vi "Door Poka Yoke_UI.vi"(8 "error in (no error)":errorcluster, 10 "Door Poka Yoke":bool, 11 "JSON FilePath":path) -> (0 "error out":errorcluster)   [LabVIEW 2019, in "ZenGage v3.0 UI.lvclass"]
uses:
  ZenGage v3.0 UI.lvclass
panel:
  out "Time taken":u32
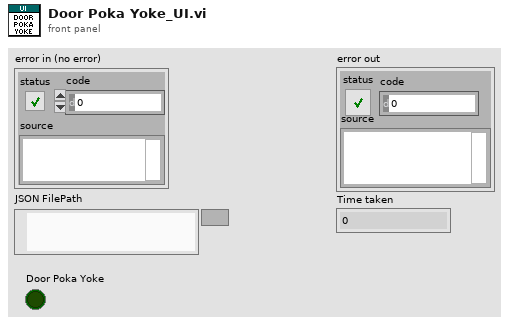
[diagram p1: front panel]
types:
  T1 = enum16{"Action Failed", "Append", "Insert", "Replace"}
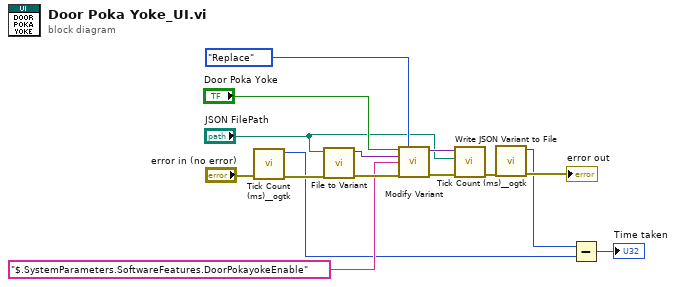
[diagram p0: block diagram]
diagram:
  n1 = call <userlib>:"Tick Count (ms)__ogtk.vi"("error in (no error)"="error in (no error)") -> ("error out"=w6:errorcluster, "millisecond timer value"=w2:u32)  [unwired: 9 in]
  n2 = call <vilib>:"File to Variant.vi"("JSON FilePath"="JSON FilePath", "error in (no error)"=w6) -> ("JSON Variant"=w14:variant, "error out"=w15:errorcluster)  [unwired: 6 in, 1 out]
  n3 = call <vilib>:"Modify Variant.vi"("New element in"="Door Poka Yoke", "Functionality"=T1."Replace", "Parent variant in"=w14, "JSON query path"="$.SystemParameters.SoftwareFeatures.DoorPokayokeEnable", "error in (no error)"=w15) -> ("VCluster out"=w9:variant, "error out"=w10:errorcluster)  [unwired: 6 in, 3 out]
  n4 = call <vilib>:"Write JSON Variant to File.vi"("Error In"=w10, "file (use dialog)"="JSON FilePath", "JSON Varaint"=w9) -> ("error out"=w5:errorcluster)  [unwired: 8 in]
  n5 = call <userlib>:"Tick Count (ms)__ogtk.vi"("error in (no error)"=w5) -> ("error out"=→"error out":errorcluster, "millisecond timer value"=w3:u32)  [unwired: 9 in]
  n6 = Subtract(x=w3, y=w2) -> (x-y=→"Time taken":u32)
